vi "nanocal -- nuclear schottky fit V8.vi"() -> ()   [LabVIEW 2021] (continued)
\"τ12\" -> 0.000000000000   ,  \"τ22\" -> 0.000000000000   ,  \"τN1\" -> 0.000000000000   ,  \"τN2\" -> 0.000000000000   ,  \"σηlogτ1 \" -> 0.000000000000   ,  \"σηlogτS\" -> 0.000000000000   ,  \"σηlogτN\" -> 0.000000000000   ,  \"σlogτ1\" -> 0.000000000000   ,  \"σlogτS\" -> 0.000000000000   ,  \"σlogτN\" -> 0.000000000000   ,  \"σητ1\" -> 0.000000000000   ,  \"σητS \" -> 0.000000000000   ,  \"σητN\" -> 0.000000000000    |>   , \n\"IDS0320_210901_RAW_cal__ref_\" ->   <|    \"ζ\" -> 0.020503230875   ,  \"τ1\" -> 0.009039124549   ,  \"τS\" -> 0.020793619650   ,  \"τN\" -> 0.000681175648   ,  \"τC\" -> 0.003316390430   ,  \"κ0\" -> 0.000000005460   ,  \"mm1\" -> 0.000057758980   ,  \"mm2\" -> 0.008659022853   ,  \"mm3\" -> 0.025553831130   ,  \"T\" -> 0.830000000000   ,  \"B\" -> 12.000000000000   ,  \"θ\" -> 45.000000000000   ,  \"Reoff\" -> 0.000000000000   ,  \"Imoff\" -> 0.000000000000   ,  \"στ1\" -> 0.000055900109   ,  \"στS\" -> 0.000001990468   ,  \"στN\" -> 0.000002087760   ,  \"τ11 \" -> 0.000000000000   ,  \"τ12\" -> 0.000000000000   ,  \"τ22\" -> 0.000000000000   ,  \"τN1\" -> 0.000000000000   ,  \"τN2\" -> 0.000000000000   ,  \"σηlogτ1 \" -> 0.065405279709   ,  \"σηlogτS\" -> 0.000181229469   ,  \"σηlogτN\" -> 0.048239068739   ,  \"σlogτ1\" -> 0.006184239243   ,  \"σlogτS\" -> 0.000095724945   ,  \"σlogτN\" -> 0.003064936921   ,  \"σητ1\" -> 0.000591206469   ,  \"σητS \" -> 0.000003768417   ,  \"σητN\" -> 0.000032859279    |>   , \n\"IDS0320_210901_RAW_cal__sam_\" ->   <|    \"ζ\" -> 0.023591124045   ,  \"τ1\" -> 0.014910006225   ,  \"τS\" -> 0.019342950404   ,  \"τN\" -> 0.000752972387   ,  \"τC\" -> 0.004900413232   ,  \"κ0\" -> 0.000000005453   ,  \"mm1\" -> 0.000090864236   ,  \"mm2\" -> 0.013909604856   ,  \"mm3\" -> 0.026379958563   ,  \"T\" -> 0.830000000000   ,  \"B\" -> 12.000000000000   ,  \"θ\" -> 45.000000000000   ,  \"Reoff\" -> 0.000000000000   ,  \"Imoff\" -> 0.000000000000   ,  \"στ1\" -> 0.000000000000   ,  \"στS\" -> 0.000000000000   ,  \"στN\" -> 0.000000000000   ,  \"τ11 \" -> 0.000000000000   ,  \"τ12\" -> 0.000000000000   ,  \"τ22\" -> 0.000000000000   ,  \"τN1\" -> 0.000000000000   ,  \"τN2\" -> 0.000000000000   ,  \"σηlogτ1 \" -> 0.000000000000   ,  \"σηlogτS\" -> 0.000000000000   ,  \"σηlogτN\" -> 0.000000000000   ,  \"σlogτ1\" -> 0.000000000000   ,  \"σlogτS\" -> 0.000000000000   ,  \"σlogτN\" -> 0.000000000000   ,  \"σητ1\" -> 0.000000000000   ,  \"σητS \" -> 0.000000000000   ,  \"σητN\" -> 0.000000000000    |>   , \n\"IDS0321_210901_RAW_cal__ref_\" ->   <|    \"ζ\" -> 0.017045320784   ,  \"τ1\" -> 0.008431183859   ,  \"τS\" -> 0.017976343705   ,  \"τN\" -> 0.000325056169   ,  \"τC\" -> 0.003125498952   ,  \"κ0\" -> 0.000000007605   ,  \"mm1\" -> 0.000044827954   ,  \"mm2\" -> 0.008224435737   ,  \"mm3\" -> 0.021900772225   ,  \"T\" -> 1.130000000000   ,  \"B\" -> 12.000000000000   ,  \"θ\" -> 45.000000000000   ,  \"Reoff\" -> 0.000000000000   ,  \"Imoff\" -> 0.000000000000   ,  \"στ1\" -> 0.000106874895   ,  \"στS\" -> 0.000001909550   ,  \"στN\" -> 0.000002033159   ,  \"τ11 \" -> 0.000000000000   ,  \"τ12\" -> 0.000000000000   ,  \"τ22\" -> 0.000000000000   ,  \"τN1\" -> 0.000000000000   ,  \"τN2\" -> 0.000000000000   ,  \"σηlogτ1 \" -> 0.062850108994   ,  \"σηlogτS\" -> 0.000092098148   ,  \"σηlogτN\" -> 0.047786050692   ,  \"σlogτ1\" -> 0.012676143384   ,  \"σlogτS\" -> 0.000106225712   ,  \"σlogτN\" -> 0.006254792961   ,  \"σητ1\" -> 0.000529900824   ,  \"σητS \" -> 0.000001655588   ,  \"σητN\" -> 0.000015533151    |>   , \n\"IDS0321_210901_RAW_cal__sam_\" ->   <|    \"ζ\" -> 0.020215154826   ,  \"τ1\" -> 0.014105227254   ,  \"τS\" -> 0.015660924043   ,  \"τN\" -> 0.000525137036   ,  \"τC\" -> 0.005447728357   ,  \"κ0\" -> 0.000000007594   ,  \"mm1\" -> 0.000080798630   ,  \"mm2\" -> 0.013233003317   ,  \"mm3\" -> 0.022752418474   ,  \"T\" -> 1.130000000000   ,  \"B\" -> 12.000000000000   ,  \"θ\" -> 45.000000000000   ,  \"Reoff\" -> 0.000000000000   ,  \"Imoff\" -> 0.000000000000   ,  \"στ1\" -> 0.000000000000   ,  \"στS\" -> 0.000000000000   ,  \"στN\" -> 0.000000000000   ,  \"τ11 \" -> 0.000000000000   ,  \"τ12\" -> 0.000000000000   ,  \"τ22\" -> 0.000000000000   ,  \"τN1\" -> 0.000000000000   ,  \"τN2\" -> 0.000000000000   ,  \"σηlogτ1 \" -> 0.000000000000   ,  \"σηlogτS\" -> 0.000000000000   ,  \"σηlogτN\" -> 0.000000000000   ,  \"σlogτ1\" -> 0.000000000000   ,  \"σlogτS\" -> 0.000000000000   ,  \"σlogτN\" -> 0.000000000000   ,  \"σητ1\" -> 0.000000000000   ,  \"σητS \" -> 0.000000000000   ,  \"σητN\" -> 0.000000000000    |>   , \n\"IDS0322_210901_RAW_cal__ref_\" ->   <|    \"ζ\" -> 0.013563339725   ,  \"τ1\" -> 0.010588752100   ,  \"τS\" -> 0.012516826904   ,  \"τN\" -> 0.000053088444   ,  \"τC\" -> 0.003706516858   ,  \"κ0\" -> 0.000000013118   ,  \"mm1\" -> 0.000038475513   ,  \"mm2\" -> 0.010492542946   ,  \"mm3\" -> 0.016504655879   ,  \"T\" -> 1.900000000000   ,  \"B\" -> 12.000000000000   ,  \"θ\" -> 45.000000000000   ,  \"Reoff\" -> 0.000000000000   ,  \"Imoff\" -> 0.000000000000   ,  \"στ1\" -> 0.000668754885   ,  \"στS\" -> 0.000001256386   ,  \"στN\" -> 0.000001711917   ,  \"τ11 \" -> 0.000000000000   ,  \"τ12\" -> 0.000000000000   ,  \"τ22\" -> 0.000000000000   ,  \"τN1\" -> 0.000000000000   ,  \"τN2\" -> 0.000000000000   ,  \"σηlogτ1 \" -> 0.046872894562   ,  \"σηlogτS\" -> 0.000010676949   ,  \"σηlogτN\" -> 0.045178485775   ,  \"σlogτ1\" -> 0.063157100934   ,  \"σlogτS\" -> 0.000100375785   ,  \"σlogτN\" -> 0.032246499932   ,  \"σητ1\" -> 0.000496325461   ,  \"σητS \" -> 0.000000133642   ,  \"σητN\" -> 0.000002398456    |>   , \n\"IDS0322_210901_RAW_cal__sam_\" ->   <|    \"ζ\" -> 0.018090572724   ,  \"τ1\" -> 0.013314780956   ,  \"τS\" -> 0.010820835010   ,  \"τN\" -> 0.000265552167   ,  \"τC\" -> 0.005393540417   ,  \"κ0\" -> 0.000000013100   ,  \"mm1\" -> 0.000064590824   ,  \"mm2\" -> 0.012452255889   ,  \"mm3\" -> 0.017478420931   ,  \"T\" -> 1.900000000000   ,  \"B\" -> 12.000000000000   ,  \"θ\" -> 45.000000000000   ,  \"Reoff\" -> 0.000000000000   ,  \"Imoff\" -> 0.000000000000   ,  \"στ1\" -> 0.000000000000   ,  \"στS\" -> 0.000000000000   ,  \"στN\" -> 0.000000000000   ,  \"τ11 \" -> 0.000000000000   ,  \"τ12\" -> 0.000000000000   ,  \"τ22\" -> 0.000000000000   ,  \"τN1\" -> 0.000000000000   ,  \"τN2\" -> 0.000000000000   ,  \"σηlogτ1 \" -> 0.000000000000   ,  \"σηlogτS\" -> 0.000000000000   ,  \"σηlogτN\" -> 0.000000000000   ,  \"σlogτ1\" -> 0.000000000000   ,  \"σlogτS\" -> 0.000000000000   ,  \"σlogτN\" -> 0.000000000000   ,  \"σητ1\" -> 0.000000000000   ,  \"σητS \" -> 0.000000000000   ,  \"σητN\" -> 0.000000000000    |>   , \n\"IDS0323_210901_RAW_cal__ref_\" ->   <|    \"ζ\" -> 0.018293099786   ,  \"τ1\" -> 0.011708031233   ,  \"τS\" -> 0.007423574930   ,  \"τN\" -> 0.000011193776   ,  \"τC\" -> 0.004650795843   ,  \"κ0\" -> 0.000000023552   ,  \"mm1\" -> 0.000051946515   ,  \"mm2\" -> 0.011507133440   ,  \"mm3\" -> 0.012370520793   ,  \"T\" -> 3.100000000000   ,  \"B\" -> 12.000000000000   ,  \"θ\" -> 45.000000000000   ,  \"Reoff\" -> 0.000000000000   ,  \"Imoff\" -> 0.000000000000   ,  \"στ1\" -> 0.475647244470   ,  \"στS\" -> 0.000355048882   ,  \"στN\" -> 0.206336535576   ,  \"τ11 \" -> 0.000000000000   ,  \"τ12\" -> 0.000000000000   ,  \"τ22\" -> 0.000000000000   ,  \"τN1\" -> 0.000000000000   ,  \"τN2\" -> 0.000000000000   ,  \"σηlogτ1 \" -> 0.000000000000   ,  \"σηlogτS\" -> 0.000000000000   ,  \"σηlogτN\" -> 0.000000000000   ,  \"σlogτ1\" -> 0.000000000000   ,  \"σlogτS\" -> 0.000000000000   ,  \"σlogτN\" -> 0.000000000000   ,  \"σητ1\" -> 0.000000000000   ,  \"σητS \" -> 0.000000000000   ,  \"σητN\" -> 0.000000000000    |>   , \n\"IDS0323_210901_RAW_cal__sam_\" ->   <|    \"ζ\" -> 0.019438138135   ,  \"τ1\" -> 0.013521019406   ,  \"τS\" -> 0.007253169401   ,  \"τN\" -> 0.000154824830   ,  \"τC\" -> 0.004746579385   ,  \"κ0\" -> 0.000000023466   ,  \"mm1\" -> 0.000055371802   ,  \"mm2\" -> 0.011289401344   ,  \"mm3\" -> 0.014474817491   ,  \"T\" -> 3.100000000000   ,  \"B\" -> 12.000000000000   ,  \"θ\" -> 45.000000000000   ,  \"Reoff\" -> 0.000000000000   ,  \"Imoff\" -> 0.000000000000   ,  \"στ1\" -> 0.000000000000   ,  \"στS\" -> 0.000000000000   ,  \"στN\" -> 0.000000000000   ,  \"τ11 \" -> 0.000000000000   ,  \"τ12\" -> 0.000000000000   ,  \"τ22\" -> 0.000000000000   ,  \"τN1\" -> 0.000000000000   ,  \"τN2\" -> 0.000000000000   ,  \"σηlogτ1 \" -> 0.000000000000   ,  \"σηlogτS\" -> 0.000000000000   ,  \"σηlogτN\" -> 0.000000000000   ,  \"σlogτ1\" -> 0.000000000000   ,  \"σlogτS\" -> 0.000000000000   ,  \"σlogτN\" -> 0.000000000000   ,  \"σητ1\" -> 0.000000000000   ,  \"σητS \" -> 0.000000000000   ,  \"σητN\" -> 0.000000000000    |>   , \n\"IDS0324_210901_RAW_cal__ref_\" ->   <|    \"ζ\" -> 0.016347935479   ,  \"τ1\" -> 0.012470259059   ,  \"τS\" -> 0.004816019887   ,  \"τN\" -> 0.000001431153   ,  \"τC\" -> 0.003222477919   ,  \"κ0\" -> 0.000000058396   ,  \"mm1\" -> 0.000031377273   ,  \"mm2\" -> 0.008083179313   ,  \"mm3\" -> 0.012474386811   ,  \"T\" -> 5.700000000000   ,  \"B\" -> 12.000000000000   ,  \"θ\" -> 45.000000000000   ,  \"Reoff\" -> 0.000000000000   ,  \"Imoff\" -> 0.000000000000   ,  \"στ1\" -> 6.524200560783   ,  \"στS\" -> 0.000699627106   ,  \"στN\" -> 3.198245893215   ,  \"τ11 \" -> 0.000000000000   ,  \"τ12\" -> 0.000000000000   ,  \"τ22\" -> 0.000000000000   ,  \"τN1\" -> 0.000000000000   ,  \"τN2\" -> 0.000000000000   ,  \"σηlogτ1 \" -> 0.000000000000   ,  \"σηlogτS\" -> 0.000000000000   ,  \"σηlogτN\" -> 0.000000000000   ,  \"σlogτ1\" -> 0.000000000000   ,  \"σlogτS\" -> 0.000000000000   ,  \"σlogτN\" -> 0.000000000000   ,  \"σητ1\" -> 0.000000000000   ,  \"σητS \" -> 0.000000000000   ,  \"σητN\" -> 0.000000000000    |>   , \n\"IDS0324_210901_RAW_cal__sam_\" ->   <|    \"ζ\" -> 0.018573189054   ,  \"τ1\" -> 0.013304612245   ,  \"τS\" -> 0.003723860844   ,  \"τN\" -> 0.000084829442   ,  \"τC\" -> 0.004309703632   ,  \"κ0\" -> 0.000000058362   ,  \"mm1\" -> 0.000036954445   ,  \"mm2\" -> 0.007938616076   ,  \"mm3\" -> 0.013518175167   ,  \"T\" -> 5.700000000000   ,  \"B\" -> 12.000000000000   ,  \"θ\" -> 45.000000000000   ,  \"Reoff\" -> 0.000000000000   ,  \"Imoff\" -> 0.000000000000   ,  \"στ1\" -> 0.000000000000   ,  \"στS\" -> 0.000000000000   ,  \"στN\" -> 0.000000000000   ,  \"τ11 \" -> 0.000000000000   ,  \"τ12\" -> 0.000000000000   ,  \"τ22\" -> 0.000000000000   ,  \"τN1\" -> 0.000000000000   ,  \"τN2\" -> 0.000000000000   ,  \"σηlogτ1 \" -> 0.000000000000   ,  \"σηlogτS\" -> 0.000000000000   ,  \"σηlogτN\" -> 0.000000000000   ,  \"σlogτ1\" -> 0.000000000000   ,  \"σlogτS\" -> 0.000000000000   ,  \"σlogτN\" -> 0.000000000000   ,  \"σητ1\" -> 0.000000000000   ,  \"σητS \" -> 0.000000000000   ,  \"σητN\" -> 0.000000000000    |>   , \n\"IDS0330_210901_RAW_cal__ref_\" ->   <|    \"ζ\" -> 0.000000000000   ,  \"τ1\" -> 0.000000000000   ,  \"τS\" -> 0.000000000000   ,  \"τN\" -> 0.000000000000   ,  \"τC\" -> 0.000000000000   ,  \"κ0\" -> 0.000000000000   ,  \"mm1\" -> 0.000000000000   ,  \"mm2\" -> 0.000000000000   ,  \"mm3\" -> 0.000000000000   ,  \"T\" -> 0.197000000000   ,  \"B\" -> 1.000000000000   ,  \"θ\" -> 90.000000000000   ,  \"Reoff\" -> 0.000000000000   ,  \"Imoff\" -> 0.000000000000   ,  \"στ1\" -> 0.000000000000   ,  \"στS\" -> 0.000000000000   ,  \"στN\" -> 0.000000000000   ,  \"τ11 \" -> 0.000000000000   ,  \"τ12\" -> 0.000000000000   ,  \"τ22\" -> 0.000000000000   ,  \"τN1\" -> 0.000000000000   ,  \"τN2\" -> 0.000000000000   ,  \"σηlogτ1 \" -> 0.000000000000   ,  \"σηlogτS\" -> 0.000000000000   ,  \"σηlogτN\" -> 0.000000000000   ,  \"σlogτ1\" -> 0.000000000000   ,  \"σlogτS\" -> 0.000000000000   ,  \"σlogτN\" -> 0.000000000000   ,  \"σητ1\" -> 0.000000000000   ,  \"σητS \" -> 0.000000000000   ,  \"σητN\" -> 0.000000000000    |>   , \n\"IDS0330_210901_RAW_cal__sam_\" ->   <|    \"ζ\" -> 0.000000000000   ,  \"τ1\" -> 0.000000000000   ,  \"τS\" -> 0.000000000000   ,  \"τN\" -> 0.000000000000   ,  \"τC\" -> 0.000000000000   ,  \"κ0\" -> 0.000000000000   ,  \"mm1\" -> 0.000000000000   ,  \"mm2\" -> 0.000000000000   ,  \"mm3\" -> 0.000000000000   ,  \"T\" -> 0.197000000000   ,  \"B\" -> 1.000000000000   ,  \"θ\" -> 90.000000000000   ,  \"Reoff\" -> 0.000000000000   ,  \"Imoff\" -> 0.000000000000   ,  \"στ1\" -> 0.000000000000   ,  \"στS\" -> 0.000000000000   ,  \"στN\" -> 0.000000000000   ,  \"τ11 \" -> 0.000000000000   ,  \"τ12\" -> 0.000000000000   ,  \"τ22\" -> 0.000000000000   ,  \"τN1\" -> 0.000000000000   ,  \"τN2\" -> 0.000000000000   ,  \"σηlogτ1 \" -> 0.000000000000   ,  \"σηlogτS\" -> 0.000000000000   ,  \"σηlogτN\" -> 0.000000000000   ,  \"σlogτ1\" -> 0.000000000000   ,  \"σlogτS\" -> 0.000000000000   ,  \"σlogτN\" -> 0.000000000000   ,  \"σητ1\" -> 0.000000000000   ,  \"σητS \" -> 0.000000000000   ,  \"σητN\" -> 0.000000000000    |>   , \n\"IDS0331_210901_RAW_cal__ref_\" ->   <|    \"ζ\" -> 0.000000000000   ,  \"τ1\" -> 0.000000000000   ,  \"τS\" -> 0.000000000000   ,  \"τN\" -> 0.000000000000   ,  \"τC\" -> 0.000000000000   ,  \"κ0\" -> 0.000000000000   ,  \"mm1\" -> 0.000000000000   ,  \"mm2\" -> 0.000000000000   ,  \"mm3\" -> 0.000000000000   ,  \"T\" -> 0.197000000000   ,  \"B\" -> 2.000000000000   ,  \"θ\" -> 90.000000000000   ,  \"Reoff\" -> 0.000000000000   ,  \"Imoff\" -> 0.000000000000   ,  \"στ1\" -> 0.000000000000   ,  \"στS\" -> 0.000000000000   ,  \"στN\" -> 0.000000000000   ,  \"τ11 \" -> 0.000000000000   ,  \"τ12\" -> 0.000000000000   ,  \"τ22\" -> 0.000000000000   ,  \"τN1\" -> 0.000000000000   ,  \"τN2\" -> 0.000000000000   ,  \"σηlogτ1 \" -> 0.000000000000   ,  \"σηlogτS\" -> 0.000000000000   ,  \"σηlogτN\" -> 0.000000000000   ,  \"σlogτ1\" -> 0.000000000000   ,  \"σlogτS\" -> 0.000000000000   ,  \"σlogτN\" -> 0.000000000000   ,  \"σητ1\" -> 0.000000000000   ,  \"σητS \" -> 0.000000000000   ,  \"σητN\" -> 0.000000000000    |>   , \n\"IDS0331_210901_RAW_cal__sam_\" ->   <|    \"ζ\" -> 0.000000000000   ,  \"τ1\" -> 0.000000000000   ,  \"τS\" -> 0.000000000000   ,  \"τN\" -> 0.000000000000   ,  \"τC\" -> 0.000000000000   ,  \"κ0\" -> 0.000000000000   ,  \"mm1\" -> 0.000000000000   ,  \"mm2\" -> 0.000000000000   ,  \"mm3\" -> 0.000000000000   ,  \"T\" -> 0.197000000000   ,  \"B\" -> 2.000000000000   ,  \"θ\" -> 90.000000000000   ,  \"Reoff\" -> 0.000000000000   ,  \"Imoff\" -> 0.000000000000   ,  \"στ1\" -> 0.000000000000   ,  \"στS\" -> 0.000000000000   ,  \"στN\" -> 0.000000000000   ,  \"τ11 \" -> 0.000000000000   ,  \"τ12\" -> 0.000000000000   ,  \"τ22\" -> 0.000000000000   ,  \"τN1\" -> 0.000000000000   ,  \"τN2\" -> 0.000000000000   ,  \"σηlogτ1 \" -> 0.000000000000   ,  \"σηlogτS\" -> 0.000000000000   ,  \"σηlogτN\" -> 0.000000000000   ,  \"σlogτ1\" -> 0.000000000000   ,  \"σlogτS\" -> 0.000000000000   ,  \"σlogτN\" -> 0.000000000000   ,  \"σητ1\" -> 0.000000000000   ,  \"σητS \" -> 0.000000000000   ,  \"σητN\" -> 0.000000000000    |>   , \n\"IDS0335_210904_RAW_cal__ref_\" ->   <|    \"ζ\" -> 0.207532583304   ,  \"τ1\" -> 0.025125097588   ,  \"τS\" -> 0.082589564829   ,  \"τN\" -> 0.011731487107   ,  \"τC\" -> 0.000983545190   ,  \"κ0\" -> 0.000000001029   ,  \"mm1\" -> 0.000167664032   ,  \"mm2\" -> 0.021314422468   ,  \"mm3\" -> 0.118522299782   ,  \"T\" -> 0.197000000000   ,  \"B\" -> 5.000000000000   ,  \"θ\" -> 90.000000000000   ,  \"Reoff\" -> 0.000000000000   ,  \"Imoff\" -> 0.000000000000   ,  \"στ1\" -> 0.000233587721   ,  \"στS\" -> 0.000055131581   ,  \"στN\" -> 0.000056029028   ,  \"τ11 \" -> 0.000000000000   ,  \"τ12\" -> 0.000000000000   ,  \"τ22\" -> 0.000000000000   ,  \"τN1\" -> 0.000000000000   ,  \"τN2\" -> 0.000000000000   ,  \"σηlogτ1 \" -> 0.240135972474   ,  \"σηlogτS\" -> 0.003377698192   ,  \"σηlogτN\" -> 0.153140041107   ,  \"σlogτ1\" -> 0.009296987616   ,  \"σlogτS\" -> 0.000667536885   ,  \"σlogτN\" -> 0.004775952743   ,  \"σητ1\" -> 0.006033439743   ,  \"σητS \" -> 0.000278962624   ,  \"σητN\" -> 0.001796560418    |>   , \n\"IDS0335_210904_RAW_cal__sam_\" ->   <|    \"ζ\" -> 0.127476550533   ,  \"τ1\" -> 0.026692349363   ,  \"τS\" -> 0.111739634553   ,  \"τN\" -> 0.012149249884   ,  \"τC\" -> 0.001469649387   ,  \"κ0\" -> 0.000000001130   ,  \"mm1\" -> 0.000164458900   ,  \"mm2\" -> 0.023578369229   ,  \"mm3\" -> 0.144100982695   ,  \"T\" -> 0.197000000000   ,  \"B\" -> 5.000000000000   ,  \"θ\" -> 90.000000000000   ,  \"Reoff\" -> -19117469.879518091700   ,  \"Imoff\" -> 0.000000000000   ,  \"στ1\" -> 0.000000000000   ,  \"στS\" -> 0.000000000000   ,  \"στN\" -> 0.000000000000   ,  \"τ11 \" -> 0.000000000000   ,  \"τ12\" -> 0.000000000000   ,  \"τ22\" -> 0.000000000000   ,  \"τN1\" -> 0.000000000000   ,  \"τN2\" -> 0.000000000000   ,  \"σηlogτ1 \" -> 0.000000000000   ,  \"σηlogτS\" -> 0.000000000000   ,  \"σηlogτN\" -> 0.000000000000   ,  \"σlogτ1\" -> 0.000000000000   ,  \"σlogτS\" -> 0.000000000000   ,  \"σlogτN\" -> 0.000000000000   ,  \"σητ1\" -> 0.000000000000   ,  \"σητS \" -> 0.000000000000   ,  \"σητN\" -> 0.000000000000    |>   , \n\"IDS0336_210904_RAW_cal__ref_\" ->   <|    \"ζ\" -> 0.404996144537   ,  \"τ1\" -> 0.024160753157   ,  \"τS\" -> 0.156601011699   ,  \"τN\" -> 0.067300002147   ,  \"τC\" -> 0.001060374872   ,  \"κ0\" -> 0.000000000386   ,  \"mm1\" -> 0.000304605514   ,  \"mm2\" -> 0.016515851644   ,  \"mm3\" -> 0.322980732083   ,  \"T\" -> 0.122000000000   ,  \"B\" -> 5.000000000000   ,  \"θ\" -> 90.000000000000   ,  \"Reoff\" -> 0.000000000000   ,  \"Imoff\" -> 0.000000000000   ,  \"στ1\" -> 0.000862354049   ,  \"στS\" -> 0.001247330744   ,  \"στN\" -> 0.001270513602   ,  \"τ11 \" -> 0.000000000000   ,  \"τ12\" -> 0.000000000000   ,  \"τ22\" -> 0.000000000000   ,  \"τN1\" -> 0.000000000000   ,  \"τN2\" -> 0.000000000000   ,  \"σηlogτ1 \" -> 0.325498125549   ,  \"σηlogτS\" -> 0.015432787187   ,  \"σηlogτN\" -> 0.180441177358   ,  \"σlogτ1\" -> 0.035692349629   ,  \"σlogτS\" -> 0.007965023540   ,  \"σlogτN\" -> 0.018878359005   ,  \"σητ1\" -> 0.007864279864   ,  \"σητS \" -> 0.002416790087   ,  \"σητN\" -> 0.012143691624    |>   , \n\"IDS0336_210904_RAW_cal__sam_\" ->   <|    \"ζ\" -> 0.192483765517   ,  \"τ1\" -> 0.038218926206   ,  \"τS\" -> 0.302700165376   ,  \"τN\" -> 0.092288910100   ,  \"τC\" -> 0.001788727736   ,  \"κ0\" -> 0.000000000500   ,  \"mm1\" -> 0.000287527431   ,  \"mm2\" -> 0.028741269140   ,  \"mm3\" -> 0.481996917433   ,  \"T\" -> 0.122000000000   ,  \"B\" -> 5.000000000000   ,  \"θ\" -> 90.000000000000   ,  \"Reoff\" -> 0.000000000000   ,  \"Imoff\" -> 0.000000000000   ,  \"στ1\" -> 0.000000000000   ,  \"στS\" -> 0.000000000000   ,  \"στN\" -> 0.000000000000   ,  \"τ11 \" -> 0.000000000000   ,  \"τ12\" -> 0.000000000000   ,  \"τ22\" -> 0.000000000000   ,  \"τN1\" -> 0.000000000000   ,  \"τN2\" -> 0.000000000000   ,  \"σηlogτ1 \" -> 0.000000000000   ,  \"σηlogτS\" -> 0.000000000000   ,  \"σηlogτN\" -> 0.000000000000   ,  \"σlogτ1\" -> 0.000000000000   ,  \"σlogτS\" -> 0.000000000000   ,  \"σlogτN\" -> 0.000000000000   ,  \"σητ1\" -> 0.000000000000   ,  \"σητS \" -> 0.000000000000   ,  \"σητN\" -> 0.000000000000    |>   , \n\"IDS0337_210904_RAW_cal__ref_\" ->   <|    \"ζ\" -> 0.297990585942   ,  \"τ1\" -> 0.031304623149   ,  \"τS\" -> 0.124641982645   ,  \"τN\" -> 0.023046606001   ,  \"τC\" -> 0.000944607794   ,  \"κ0\" -> 0.000000000638   ,  \"mm1\" -> 0.000215887866   ,  \"mm2\" -> 0.025688492755   ,  \"mm3\" -> 0.198043248034   ,  \"T\" -> 0.157000000000   ,  \"B\" -> 5.000000000000   ,  \"θ\" -> 90.000000000000   ,  \"Reoff\" -> 0.000000000000   ,  \"Imoff\" -> 0.000000000000   ,  \"στ1\" -> 0.000567275610   ,  \"στS\" -> 0.000219510526   ,  \"στN\" -> 0.000220252373   ,  \"τ11 \" -> 0.000000000000   ,  \"τ12\" -> 0.000000000000   ,  \"τ22\" -> 0.000000000000   ,  \"τN1\" -> 0.000000000000   ,  \"τN2\" -> 0.000000000000   ,  \"σηlogτ1 \" -> 0.272787417026   ,  \"σηlogτS\" -> 0.005452152136   ,  \"σηlogτN\" -> 0.159578496904   ,  \"σlogτ1\" -> 0.018121144825   ,  \"σlogτS\" -> 0.001761128324   ,  \"σlogτN\" -> 0.009556824666   ,  \"σητ1\" -> 0.008539507290   ,  \"σητS \" -> 0.000679567052   ,  \"σητN\" -> 0.003677742744    |>   , \n\"IDS0337_210904_RAW_cal__sam_\" ->   <|    \"ζ\" -> 0.174989526301   ,  \"τ1\" -> 0.032277116931   ,  \"τS\" -> 0.156061636315   ,  \"τN\" -> 0.033861256896   ,  \"τC\" -> 0.001461638306   ,  \"κ0\" -> 0.000000000742   ,  \"mm1\" -> 0.000216209109   ,  \"mm2\" -> 0.025810900049   ,  \"mm3\" -> 0.230869056407   ,  \"T\" -> 0.157000000000   ,  \"B\" -> 5.000000000000   ,  \"θ\" -> 90.000000000000   ,  \"Reoff\" -> -41753012.048192769300   ,  \"Imoff\" -> 0.000000000000   ,  \"στ1\" -> 0.000000000000   ,  \"στS\" -> 0.000000000000   ,  \"στN\" -> 0.000000000000   ,  \"τ11 \" -> 0.000000000000   ,  \"τ12\" -> 0.000000000000   ,  \"τ22\" -> 0.000000000000   ,  \"τN1\" -> 0.000000000000   ,  \"τN2\" -> 0.000000000000   ,  \"σηlogτ1 \" -> 0.000000000000   ,  \"σηlogτS\" -> 0.000000000000   ,  \"σηlogτN\" -> 0.000000000000   ,  \"σlogτ1\" -> 0.000000000000   ,  \"σlogτS\" -> 0.000000000000   ,  \"σlogτN\" -> 0.000000000000   ,  \"σητ1\" -> 0.000000000000   ,  \"σητS \" -> 0.000000000000   ,  \"σητN\" -> 0.000000000000    |>   , \n\"IDS0338_210904_RAW_cal__ref_\" ->   <|    \"ζ\" -> 0.265658527884   ,  \"τ1\" -> 0.023120075726   ,  \"τS\" -> 0.103313442466   ,  \"τN\" -> 0.020697464258   ,  \"τC\" -> 0.000912229768   ,  \"κ0\" -> 0.000000000737   ,  \"mm1\" -> 0.000190421821   ,  \"mm2\" -> 0.018760460104   ,  \"mm3\" -> 0.162036885215   ,  \"T\" -> 0.170000000000   ,  \"B\" -> 5.000000000000   ,  \"θ\" -> 90.000000000000   ,  \"Reoff\" -> 0.000000000000   ,  \"Imoff\" -> 0.000000000000   ,  \"στ1\" -> 0.000288316469   ,  \"στS\" -> 0.000137331811   ,  \"στN\" -> 0.000137381757   ,  \"τ11 \" -> 0.000000000000   ,  \"τ12\" -> 0.000000000000   ,  \"τ22\" -> 0.000000000000   ,  \"τN1\" -> 0.000000000000   ,  \"τN2\" -> 0.000000000000   ,  \"σηlogτ1 \" -> 0.284385432190   ,  \"σηlogτS\" -> 0.006339746651   ,  \"σηlogτN\" -> 0.161800590932   ,  \"σlogτ1\" -> 0.012470394664   ,  \"σlogτS\" -> 0.001329273401   ,  \"σlogτN\" -> 0.006637612960   ,  \"σητ1\" -> 0.006575012728   ,  \"σητS \" -> 0.000654981051   ,  \"σητN\" -> 0.003348861948    |>   , \n\"IDS0338_210904_RAW_cal__sam_\" ->   <|    \"ζ\" -> 0.165649151389   ,  \"τ1\" -> 0.028874600848   ,  \"τS\" -> 0.141983523605   ,  \"τN\" -> 0.021766467668   ,  \"τC\" -> 0.001383503895   ,  \"κ0\" -> 0.000000000838   ,  \"mm1\" -> 0.000195205233   ,  \"mm2\" -> 0.024502619119   ,  \"mm3\" -> 0.196435318758   ,  \"T\" -> 0.170000000000   ,  \"B\" -> 5.000000000000   ,  \"θ\" -> 90.000000000000   ,  \"Reoff\" -> -35397590.361445784600   ,  \"Imoff\" -> 0.000000000000   ,  \"στ1\" -> 0.000000000000   ,  \"στS\" -> 0.000000000000   ,  \"στN\" -> 0.000000000000   ,  \"τ11 \" -> 0.000000000000   ,  \"τ12\" -> 0.000000000000   ,  \"τ22\" -> 0.000000000000   ,  \"τN1\" -> 0.000000000000   ,  \"τN2\" -> 0.000000000000   ,  \"σηlogτ1 \" -> 0.000000000000   ,  \"σηlogτS\" -> 0.000000000000   ,  \"σηlogτN\" -> 0.000000000000   ,  \"σlogτ1\" -> 0.000000000000   ,  \"σlogτS\" -> 0.000000000000   ,  \"σlogτN\" -> 0.000000000000   ,  \"σητ1\" -> 0.000000000000   ,  \"σητS \" -> 0.000000000000   ,  \"σητN\" -> 0.000000000000    |>   , \n\"IDS0339_210904_RAW_cal__ref_\" ->   <|    \"ζ\" -> 0.114039542964   ,  \"τ1\" -> 0.023293546514   ,  \"τS\" -> 0.060135025475   ,  \"τN\" -> 0.005147326644   ,  \"τC\" -> 0.001354301187   ,  \"κ0\" -> 0.000000001349   ,  \"mm1\" -> 0.000136157097   ,  \"mm2\" -> 0.020781344892   ,  \"mm3\" -> 0.076457467431   ,  \"T\" -> 0.255000000000   ,  \"B\" -> 5.000000000000   ,  \"θ\" -> 90.000000000000   ,  \"Reoff\" -> 0.000000000000   ,  \"Imoff\" -> 0.000000000000   ,  \"στ1\" -> 0.000249233332   ,  \"στS\" -> 0.000026082358   ,  \"στN\" -> 0.000027486518   ,  \"τ11 \" -> 0.000000000000   ,  \"τ12\" -> 0.000000000000   ,  \"τ22\" -> 0.000000000000   ,  \"τN1\" -> 0.000000000000   ,  \"τN2\" -> 0.000000000000   ,  \"σηlogτ1 \" -> 0.202736508629   ,  \"σηlogτS\" -> 0.001489466713   ,  \"σηlogτN\" -> 0.146001002326   ,  \"σlogτ1\" -> 0.010699673046   ,  \"σlogτS\" -> 0.000433729889   ,  \"σlogτN\" -> 0.005339959858   ,  \"σητ1\" -> 0.004722452294   ,  \"σητS \" -> 0.000089569119   ,  \"σητN\" -> 0.000751514849    |>   , \n\"IDS0339_210904_RAW_cal__sam_\" ->   <|    \"ζ\" -> 0.070510248751   ,  \"τ1\" -> 0.022152847239   ,  \"τS\" -> 0.078660981887   ,  \"τN\" -> 0.006346817462   ,  \"τC\" -> 0.001852903257   ,  \"κ0\" -> 0.000000001477   ,  \"mm1\" -> 0.000119580835   ,  \"mm2\" -> 0.020081415868   ,  \"mm3\" -> 0.094806474219   ,  \"T\" -> 0.255000000000   ,  \"B\" -> 5.000000000000   ,  \"θ\" -> 90.000000000000   ,  \"Reoff\" -> -9000000.000000000000   ,  \"Imoff\" -> 0.000000000000   ,  \"στ1\" -> 0.000000000000   ,  \"στS\" -> 0.000000000000   ,  \"στN\" -> 0.000000000000   ,  \"τ11 \" -> 0.000000000000   ,  \"τ12\" -> 0.000000000000   ,  \"τ22\" -> 0.000000000000   ,  \"τN1\" -> 0.000000000000   ,  \"τN2\" -> 0.000000000000   ,  \"σηlogτ1 \" -> 0.000000000000   ,  \"σηlogτS\" -> 0.000000000000   ,  \"σηlogτN\" -> 0.000000000000   ,  \"σlogτ1\" -> 0.000000000000   ,  \"σlogτS\" -> 0.000000000000   ,  \"σlogτN\" -> 0.000000000000   ,  \"σητ1\" -> 0.000000000000   ,  \"σητS \" -> 0.000000000000   ,  \"σητN\" -> 0.000000000000    |>   , \n\"IDS0340_210904_RAW_cal__ref_\" ->   <|    \"ζ\" -> 0.076525648542   ,  \"τ1\" -> 0.027695674574   ,  \"τS\" -> 0.050135533571   ,  \"τN\" -> 0.002521537223   ,  \"τC\" -> 0.001686073318   ,  \"κ0\" -> 0.000000001730   ,  \"mm1\" -> 0.000116467998   ,  \"mm2\" -> 0.025407303981   ,  \"mm3\" -> 0.060544663199   ,  \"T\" -> 0.308000000000   ,  \"B\" -> 5.000000000000   ,  \"θ\" -> 90.000000000000   ,  \"Reoff\" -> 0.000000000000   ,  \"Imoff\" -> 0.000000000000   ,  \"στ1\" -> 0.000231753766   ,  \"στS\" -> 0.000008787417   ,  \"στN\" -> 0.000010480438   ,  \"τ11 \" -> 0.000000000000   ,  \"τ12\" -> 0.000000000000   ,  \"τ22\" -> 0.000000000000   ,  \"τN1\" -> 0.000000000000   ,  \"τN2\" -> 0.000000000000   ,  \"σηlogτ1 \" -> 0.162472207290   ,  \"σηlogτS\" -> 0.000540904127   ,  \"σηlogτN\" -> 0.139012219140   ,  \"σlogτ1\" -> 0.008367868614   ,  \"σlogτS\" -> 0.000175273227   ,  \"σlogτN\" -> 0.004156368718   ,  \"σητ1\" -> 0.004499777380   ,  \"σητS \" -> 0.000027118517   ,  \"σητN\" -> 0.000350524485    |>   , \n\"IDS0340_210904_RAW_cal__sam_\" ->   <|    \"ζ\" -> 0.049192434897   ,  \"τ1\" -> 0.021139048522   ,  \"τS\" -> 0.064524263818   ,  \"τN\" -> 0.003413094239   ,  \"τC\" -> 0.002227810965   ,  \"κ0\" -> 0.000000001879   ,  \"mm1\" -> 0.000101271202   ,  \"mm2\" -> 0.019728994700   ,  \"mm3\" -> 0.074815955705   ,  \"T\" -> 0.308000000000   ,  \"B\" -> 5.000000000000   ,  \"θ\" -> 90.000000000000   ,  \"Reoff\" -> -4933734.939759036530   ,  \"Imoff\" -> 0.000000000000   ,  \"στ1\" -> 0.000000000000   ,  \"στS\" -> 0.000000000000   ,  \"στN\" -> 0.000000000000   ,  \"τ11 \" -> 0.000000000000   ,  \"τ12\" -> 0.000000000000   ,  \"τ22\" -> 0.000000000000   ,  \"τN1\" -> 0.000000000000   ,  \"τN2\" -> 0.000000000000   ,  \"σηlogτ1 \" -> 0.000000000000   ,  \"σηlogτS\" -> 0.000000000000   ,  \"σηlogτN\" -> 0.000000000000   ,  \"σlogτ1\" -> 0.000000000000   ,  \"σlogτS\" -> 0.000000000000   ,  \"σlogτN\" -> 0.000000000000   ,  \"σητ1\" -> 0.000000000000   ,  \"σητS \" -> 0.000000000000   ,  \"σητN\" -> 0.000000000000    |>   , \n\"IDS0341_210904_RAW_cal__ref_\" ->   <|    \"ζ\" -> 0.056782811482   ,  \"τ1\" -> 0.026331968848   ,  \"τS\" -> 0.042767805397   ,  \"τN\" -> 0.001889396139   ,  \"τC\" -> 0.002016272015   ,  \"κ0\" -> 0.000000002097   ,  \"mm1\" -> 0.000103939246   ,  \"mm2\" -> 0.024219601276   ,  \"mm3\" -> 0.051217663333   ,  \"T\" -> 0.360000000000   ,  \"B\" -> 5.000000000000   ,  \"θ\" -> 90.000000000000   ,  \"Reoff\" -> 0.000000000000   ,  \"Imoff\" -> 0.000000000000   ,  \"στ1\" -> 0.000101422442   ,  \"στS\" -> 0.000002887305   ,  \"στN\" -> 0.000003653210   ,  \"τ11 \" -> 0.000000000000   ,  \"τ12\" -> 0.000000000000   ,  \"τ22\" -> 0.000000000000   ,  \"τN1\" -> 0.000000000000   ,  \"τN2\" -> 0.000000000000   ,  \"σηlogτ1 \" -> 0.151982642430   ,  \"σηlogτS\" -> 0.000404656843   ,  \"σηlogτN\" -> 0.137111244570   ,  \"σlogτ1\" -> 0.003851684700   ,  \"σlogτS\" -> 0.000067511173   ,  \"σlogτN\" -> 0.001933533055   ,  \"σητ1\" -> 0.004002002206   ,  \"σητS \" -> 0.000017306285   ,  \"σητN\" -> 0.000259057456    |>   , \n\"IDS0341_210904_RAW_cal__sam_\" ->   <|    \"ζ\" -> 0.036062522071   ,  \"τ1\" -> 0.018116162768   ,  \"τS\" -> 0.055032833309   ,  \"τN\" -> 0.002026723445   ,  \"τC\" -> 0.002755523522   ,  \"κ0\" -> 0.000000002282   ,  \"mm1\" -> 0.000091630452   ,  \"mm2\" -> 0.017261892165   ,  \"mm3\" -> 0.062635431951   ,  \"T\" -> 0.360000000000   ,  \"B\" -> 5.000000000000   ,  \"θ\" -> 90.000000000000   ,  \"Reoff\" -> -2587349.397590361540   ,  \"Imoff\" -> 0.000000000000   ,  \"στ1\" -> 0.000000000000   ,  \"στS\" -> 0.000000000000   ,  \"στN\" -> 0.000000000000   ,  \"τ11 \" -> 0.000000000000   ,  \"τ12\" -> 0.000000000000   ,  \"τ22\" -> 0.000000000000   ,  \"τN1\" -> 0.000000000000   ,  \"τN2\" -> 0.000000000000   ,  \"σηlogτ1 \" -> 0.000000000000   ,  \"σηlogτS\" -> 0.000000000000   ,  \"σηlogτN\" -> 0.000000000000   ,  \"σlogτ1\" -> 0.000000000000   ,  \"σlogτS\" -> 0.000000000000   ,  \"σlogτN\" -> 0.000000000000   ,  \"σητ1\" -> 0.000000000000   ,  \"σητS \" -> 0.000000000000   ,  \"σητN\" -> 0.000000000000    |>   , \n\"IDS0342_210904_RAW_cal__ref_\" ->   <|    \"ζ\" -> 0.041076601022   ,  \"τ1\" -> 0.018757031155   ,  \"τS\" -> 0.035968750366   ,  \"τN\" -> 0.001085416882   ,  \"τC\" -> 0.002380872433   ,  \"κ0\" -> 0.000000002638   ,  \"mm1\" -> 0.000088519730   ,  \"mm2\" -> 0.017837018319   ,  \"mm3\" -> 0.041788592031   ,  \"T\" -> 0.438000000000   ,  \"B\" -> 5.000000000000   ,  \"θ\" -> 90.000000000000   ,  \"Reoff\" -> 0.000000000000   ,  \"Imoff\" -> 0.000000000000   ,  \"στ1\" -> 0.000064198355   ,  \"στS\" -> 0.000001597078   ,  \"στN\" -> 0.000001834209   ,  \"τ11 \" -> 0.000000000000   ,  \"τ12\" -> 0.000000000000   ,  \"τ22\" -> 0.000000000000   ,  \"τN1\" -> 0.000000000000   ,  \"τN2\" -> 0.000000000000   ,  \"σηlogτ1 \" -> 0.168171879856   ,  \"σηlogτS\" -> 0.000355670898   ,  \"σηlogτN\" -> 0.139592379603   ,  \"σlogτ1\" -> 0.003422628813   ,  \"σlogτS\" -> 0.000044401831   ,  \"σlogτN\" -> 0.001689865537   ,  \"σητ1\" -> 0.003154405190   ,  \"σητS \" -> 0.000012793038   ,  \"σητN\" -> 0.000151515925    |>   , \n\"IDS0342_210904_RAW_cal__sam_\" ->   <|    \"ζ\" -> 0.027534849374   ,  \"τ1\" -> 0.019066527741   ,  \"τS\" -> 0.046236587360   ,  \"τN\" -> 0.001227722560   ,  \"τC\" -> 0.003332461518   ,  \"κ0\" -> 0.000000002852   ,  \"mm1\" -> 0.000083583563   ,  \"mm2\" -> 0.018352322518   ,  \"mm3\" -> 0.052734315722   ,  \"T\" -> 0.438000000000   ,  \"B\" -> 5.000000000000   ,  \"θ\" -> 90.000000000000   ,  \"Reoff\" -> -1846385.542168676850   ,  \"Imoff\" -> 0.000000000000   ,  \"στ1\" -> 0.000000000000   ,  \"στS\" -> 0.000000000000   ,  \"στN\" -> 0.000000000000   ,  \"τ11 \" -> 0.000000000000   ,  \"τ12\" -> 0.000000000000   ,  \"τ22\" -> 0.000000000000   ,  \"τN1\" -> 0.000000000000   ,  \"τN2\" -> 0.000000000000   ,  \"σηlogτ1 \" -> 0.000000000000   ,  \"σηlogτS\" -> 0.000000000000   ,  \"σηlogτN\" -> 0.000000000000   ,  \"σlogτ1\" -> 0.000000000000   ,  \"σlogτS\" -> 0.000000000000   ,  \"σlogτN\" -> 0.000000000000   ,  \"σητ1\" -> 0.000000000000   ,  \"σητS \" -> 0.000000000000   ,  \"σητN\" -> 0.000000000000    |>   , \n\"IDS0343_210904_RAW_cal__ref_\" ->   <|    \"ζ\" -> 0.030668897536   ,  \"τ1\" -> 0.016422384876   ,  \"τS\" -> 0.030525750501   ,  \"τN\" -> 0.000737103869   ,  \"τC\" -> 0.002827601045   ,  \"κ0\" -> 0.000000003285   ,  \"mm1\" -> 0.000077374536   ,  \"mm2\" -> 0.015772817310   ,  \"mm3\" -> 0.035621445722   ,  \"T\" -> 0.530000000000   ,  \"B\" -> 5.000000000000   ,  \"θ\" -> 90.000000000000   ,  \"Reoff\" -> 0.000000000000   ,  \"Imoff\" -> 0.000000000000   ,  \"στ1\" -> 0.000085303275   ,  \"στS\" -> 0.000001638656   ,  \"στN\" -> 0.000001890230   ,  \"τ11 \" -> 0.000000000000   ,  \"τ12\" -> 0.000000000000   ,  \"τ22\" -> 0.000000000000   ,  \"τN1\" -> 0.000000000000   ,  \"τN2\" -> 0.000000000000   ,  \"σηlogτ1 \" -> 0.166582880232   ,  \"σηlogτS\" -> 0.000279115337   ,  \"σηlogτN\" -> 0.139234460334   ,  \"σlogτ1\" -> 0.005194329317   ,  \"σlogτS\" -> 0.000053681095   ,  \"σlogτN\" -> 0.002564401366   ,  \"σητ1\" -> 0.002735688173   ,  \"σητS \" -> 0.000008520205   ,  \"σητN\" -> 0.000102630259    |>   , \n\"IDS0343_210904_RAW_cal__sam_\" ->   <|    \"ζ\" -> 0.023098882919   ,  \"τ1\" -> 0.017709986922   ,  \"τS\" -> 0.038881575014   ,  \"τN\" -> 0.000747654909   ,  \"τC\" -> 0.003803962289   ,  \"κ0\" -> 0.000000003538   ,  \"mm1\" -> 0.000078528513   ,  \"mm2\" -> 0.017209583260   ,  \"mm3\" -> 0.044770458303   ,  \"T\" -> 0.530000000000   ,  \"B\" -> 5.000000000000   ,  \"θ\" -> 90.000000000000   ,  \"Reoff\" -> -1599397.590361446140   ,  \"Imoff\" -> 0.000000000000   ,  \"στ1\" -> 0.000000000000   ,  \"στS\" -> 0.000000000000   ,  \"στN\" -> 0.000000000000   ,  \"τ11 \" -> 0.000000000000   ,  \"τ12\" -> 0.000000000000   ,  \"τ22\" -> 0.000000000000   ,  \"τN1\" -> 0.000000000000   ,  \"τN2\" -> 0.000000000000   ,  \"σηlogτ1 \" -> 0.000000000000   ,  \"σηlogτS\" -> 0.000000000000   ,  \"σηlogτN\" -> 0.000000000000   ,  \"σlogτ1\" -> 0.000000000000   ,  \"σlogτS\" -> 0.000000000000   ,  \"σlogτN\" -> 0.000000000000   ,  \"σητ1\" -> 0.000000000000   ,  \"σητS \" -> 0.000000000000   ,  \"σητN\" -> 0.000000000000    |>   , \n\"IDS0344_210904_RAW_cal__ref_\" ->   <|    \"ζ\" -> 0.026709812446   ,  \"τ1\" -> 0.026755113102   ,  \"τS\" -> 0.027056221253   ,  \"τN\" -> 0.000433685724   ,  \"τC\" -> 0.002938863970   ,  \"κ0\" -> 0.000000003892   ,  \"mm1\" -> 0.000069295841   ,  \"mm2\" -> 0.024848155482   ,  \"mm3\" -> 0.033000682985   ,  \"T\" -> 0.620000000000   ,  \"B\" -> 5.000000000000   ,  \"θ\" -> 90.000000000000   ,  \"Reoff\" -> 0.000000000000   ,  \"Imoff\" -> 0.000000000000   ,  \"στ1\" -> 0.000318098856   ,  \"στS\" -> 0.000001623783   ,  \"στN\" -> 0.000002850113   ,  \"τ11 \" -> 0.000000000000   ,  \"τ12\" -> 0.000000000000   ,  \"τ22\" -> 0.000000000000   ,  \"τN1\" -> 0.000000000000   ,  \"τN2\" -> 0.000000000000   ,  \"σηlogτ1 \" -> 0.118559715842   ,  \"σηlogτS\" -> 0.000074397800   ,  \"σηlogτN\" -> 0.130425012097   ,  \"σlogτ1\" -> 0.011889273453   ,  \"σlogτS\" -> 0.000060015159   ,  \"σlogτN\" -> 0.006571839401   ,  \"σητ1\" -> 0.003172078607   ,  \"σητS \" -> 0.000002012923   ,  \"σητN\" -> 0.000056563466    |>   , \n\"IDS0344_210904_RAW_cal__sam_\" ->   <|    \"ζ\" -> 0.019239644947   ,  \"τ1\" -> 0.016162010817   ,  \"τS\" -> 0.033688234899   ,  \"τN\" -> 0.000426792406   ,  \"τC\" -> 0.004393456024   ,  \"κ0\" -> 0.000000004224   ,  \"mm1\" -> 0.000073664779   ,  \"mm2\" -> 0.015859557336   ,  \"mm3\" -> 0.039393633044   ,  \"T\" -> 0.620000000000   ,  \"B\" -> 5.000000000000   ,  \"θ\" -> 90.000000000000   ,  \"Reoff\" -> -1105421.686746988450   ,  \"Imoff\" -> 0.000000000000   ,  \"στ1\" -> 0.000000000000   ,  \"στS\" -> 0.000000000000   ,  \"στN\" -> 0.000000000000   ,  \"τ11 \" -> 0.000000000000   ,  \"τ12\" -> 0.000000000000   ,  \"τ22\" -> 0.000000000000   ,  \"τN1\" -> 0.000000000000   ,  \"τN2\" -> 0.000000000000   ,  \"σηlogτ1 \" -> 0.000000000000   ,  \"σηlogτS\" -> 0.000000000000   ,  \"σηlogτN\" -> 0.000000000000   ,  \"σlogτ1\" -> 0.000000000000   ,  \"σlogτS\" -> 0.000000000000   ,  \"σlogτN\" -> 0.000000000000   ,  \"σητ1\" -> 0.000000000000   ,  \"σητS \" -> 0.000000000000   ,  \"σητN\" -> 0.000000000000    |>   , \n\"IDS0346_210904_RAW_cal__ref_\" ->   <|    \"ζ\" -> 0.407818389237   ,  \"τ1\" -> 0.059098367304   ,  \"τS\" -> 0.136395388136   ,  \"τN\" -> 0.197758233370   ,  \"τC\" -> 0.001024329886   ,  \"κ0\" -> 0.000000000393   ,  \"mm1\" -> 0.000295598957   ,  \"mm2\" -> 0.022431935370   ,  \"mm3\" -> 0.507822776048   ,  \"T\" -> 0.122000000000   ,  \"B\" -> 8.000000000000   ,  \"θ\" -> 90.000000000000   ,  \"Reoff\" -> 0.000000000000   ,  \"Imoff\" -> 0.000000000000   ,  \"στ1\" -> 0.000493664169   ,  \"στS\" -> 0.000493598095   ,  \"στN\" -> 0.000812310097   ,  \"τ11 \" -> 0.000000000000   ,  \"τ12\" -> 0.000000000000   ,  \"τ22\" -> 0.000000000000   ,  \"τN1\" -> 0.000000000000   ,  \"τN2\" -> 0.000000000000   ,  \"σηlogτ1 \" -> 0.194694000050   ,  \"σηlogτS\" -> 0.012711324010   ,  \"σηlogτN\" -> 0.173317416285   ,  \"σlogτ1\" -> 0.008353262390   ,  \"σlogτS\" -> 0.003618876720   ,  \"σlogτN\" -> 0.004107591797   ,  \"σητ1\" -> 0.011506097527   ,  \"σητS \" -> 0.001733765972   ,  \"σητN\" -> 0.034274946057    |>   , \n\"IDS0346_210904_RAW_cal__sam_\" ->   <|    \"ζ\" -> 0.199267253863   ,  \"τ1\" -> 0.050205114691   ,  \"τS\" -> 0.125855812683   ,  \"τN\" -> 0.296749666016   ,  \"τC\" -> 0.001624351903   ,  \"κ0\" -> 0.000000000535   ,  \"mm1\" -> 0.000267463038   ,  \"mm2\" -> 0.014047868056   ,  \"mm3\" -> 0.544331047407   ,  \"T\" -> 0.122000000000   ,  \"B\" -> 8.000000000000   ,  \"θ\" -> 90.000000000000   ,  \"Reoff\" -> -35716867.469879508000   ,  \"Imoff\" -> 0.000000000000   ,  \"στ1\" -> 0.000000000000   ,  \"στS\" -> 0.000000000000   ,  \"στN\" -> 0.000000000000   ,  \"τ11 \" -> 0.000000000000   ,  \"τ12\" -> 0.000000000000   ,  \"τ22\" -> 0.000000000000   ,  \"τN1\" -> 0.000000000000   ,  \"τN2\" -> 0.000000000000   ,  \"σηlogτ1 \" -> 0.000000000000   ,  \"σηlogτS\" -> 0.000000000000   ,  \"σηlogτN\" -> 0.000000000000   ,  \"σlogτ1\" -> 0.000000000000   ,  \"σlogτS\" -> 0.000000000000   ,  \"σlogτN\" -> 0.000000000000   ,  \"σητ1\" -> 0.000000000000   ,  \"σητS \" -> 0.000000000000   ,  \"σητN\" -> 0.000000000000    |>   , \n\"IDS0347_210906_RAW_cal__ref_\" ->   <|    \"ζ\" -> 0.290481808635   ,  \"τ1\" -> 0.038323944120   ,  \"τS\" -> 0.067047611498   ,  \"τN\" -> 0.095881318046   ,  \"τC\" -> 0.000911015117   ,  \"κ0\" -> 0.000000000644   ,  \"mm1\" -> 0.000203389328   ,  \"mm2\" -> 0.014222650453   ,  \"mm3\" -> 0.235065739132   ,  \"T\" -> 0.157000000000   ,  \"B\" -> 8.000000000000   ,  \"θ\" -> 90.000000000000   ,  \"Reoff\" -> 0.000000000000   ,  \"Imoff\" -> 0.000000000000   ,  \"στ1\" -> 0.000081642608   ,  \"στS\" -> 0.000055996925   ,  \"στN\" -> 0.000108329720   ,  \"τ11 \" -> 0.000000000000   ,  \"τ12\" -> 0.000000000000   ,  \"τ22\" -> 0.000000000000   ,  \"τN1\" -> 0.000000000000   ,  \"τN2\" -> 0.000000000000   ,  \"σηlogτ1 \" -> 0.166799167293   ,  \"σηlogτS\" -> 0.009320651053   ,  \"σηlogτN\" -> 0.160780135489   ,  \"σlogτ1\" -> 0.002130328947   ,  \"σlogτS\" -> 0.000835181511   ,  \"σlogτN\" -> 0.001129831357   ,  \"σητ1\" -> 0.006392401967   ,  \"σητS \" -> 0.000624927391   ,  \"σητN\" -> 0.015415811306    |>   , \n\"IDS0347_210906_RAW_cal__sam_\" ->   <|    \"ζ\" -> 0.169709128246   ,  \"τ1\" -> 0.042569783210   ,  \"τS\" -> 0.096466158196   ,  \"τN\" -> 0.116379310482   ,  \"τC\" -> 0.001498996005   ,  \"κ0\" -> 0.000000000766   ,  \"mm1\" -> 0.000215022431   ,  \"mm2\" -> 0.017656553883   ,  \"mm3\" -> 0.275164490520   ,  \"T\" -> 0.157000000000   ,  \"B\" -> 8.000000000000   ,  \"θ\" -> 90.000000000000   ,  \"Reoff\" -> -35716867.469879508000   ,  \"Imoff\" -> 0.000000000000   ,  \"στ1\" -> 0.000000000000   ,  \"στS\" -> 0.000000000000   ,  \"στN\" -> 0.000000000000   ,  \"τ11 \" -> 0.000000000000   ,  \"τ12\" -> 0.000000000000   ,  \"τ22\" -> 0.000000000000   ,  \"τN1\" -> 0.000000000000   ,  \"τN2\" -> 0.000000000000   ,  \"σηlogτ1 \" -> 0.000000000000   ,  \"σηlogτS\" -> 0.000000000000   ,  \"σηlogτN\" -> 0.000000000000   ,  \"σlogτ1\" -> 0.000000000000   ,  \"σlogτS\" -> 0.000000000000   ,  \"σlogτN\" -> 0.000000000000   ,  \"σητ1\" -> 0.000000000000   ,  \"σητS \" -> 0.000000000000   ,  \"σητN\" -> 0.000000000000    |>   , \n\"IDS0348_210906_RAW_cal__ref_\" ->   <|    \"ζ\" -> 0.234564712181   ,  \"τ1\" -> 0.031261792512   ,  \"τS\" -> 0.052786157224   ,  \"τN\" -> 0.062944714793   ,  \"τC\" -> 0.000875309632   ,  \"κ0\" -> 0.000000000764   ,  \"mm1\" -> 0.000164501338   ,  \"mm2\" -> 0.012702176672
